vi "Acquisition Status.vi"(8 "error in (no error)":errorcluster, 9 "Remarks":string, 10 "Status":bool, 11 "Controller in":refnum<class "Controller.lvclass">) -> (0 "error out":errorcluster, 3 "Controller out":refnum<class "Controller.lvclass">)   [LabVIEW 2022 SP3, in "Controller.lvlib" / "Controller.lvclass"]
uses:
  Controller.lvclass
  Controller.lvclass/Controller.ctl
  UserInterface/UserInterface Messages/Log Data Msg/Log Data Msg.lvclass/Log Data Msg.ctl
  <vilib>/ActorFramework/Message Enqueuer/Message Enqueuer.lvclass/Message Enqueuer.ctl
  Read PLC-Handler Enqueuer.vi
  Read UI Enqueuer.vi
  <vilib>/ActorFramework/Message Enqueuer/Enqueue.vi
  UserInterface/UserInterface Messages/Log Data Msg/Log Data Msg.lvclass
  C:/Program Files/National Instruments/LabVIEW 2022/vi.lib/ActorFramework/Message/Message.lvclass
  PLCHandler/PLCHandler Messages/Acknowledgement Msg/Acknowledgement Msg.lvclass
  PLCHandler/PLCHandler Messages/Sleep Msg/Sleep Msg.lvclass
  <vilib>/ActorFramework/Message Priority Queue/Priority Enqueue.vi
  <vilib>/ActorFramework/Message Enqueuer/Message Enqueuer.lvclass
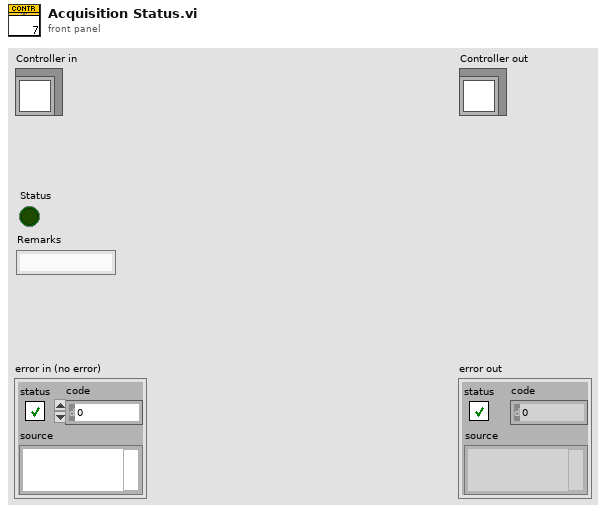
[diagram p1: front panel]
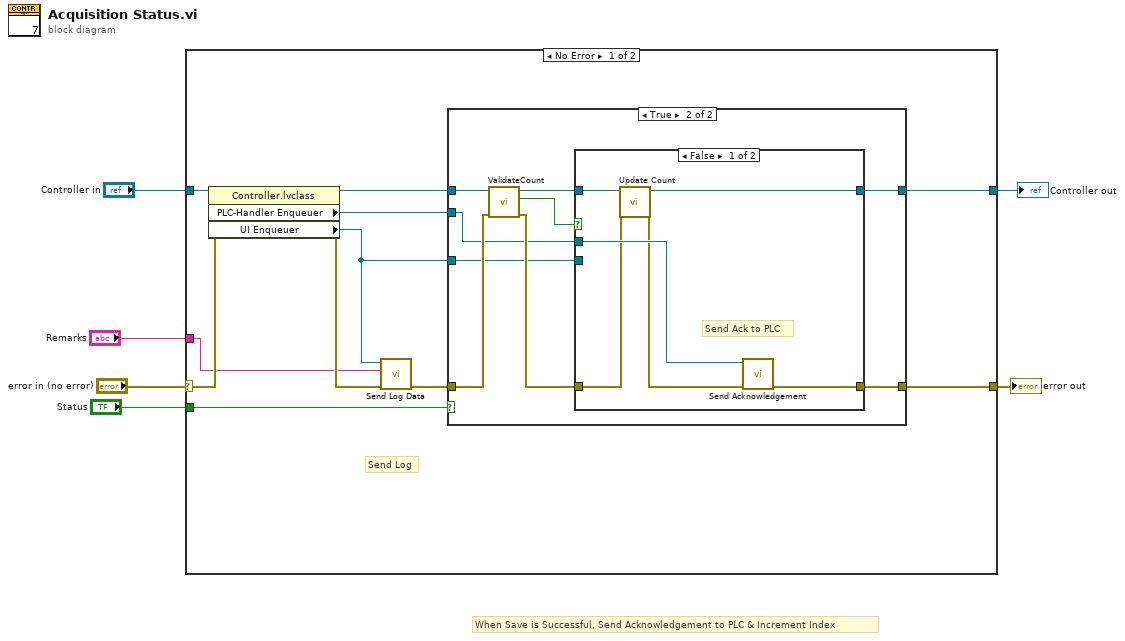
[diagram p0: block diagram]
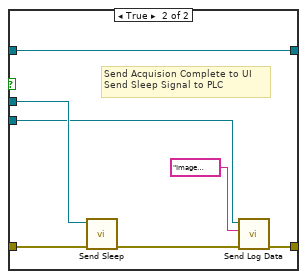
[diagram p3: hidden frame]
diagram:
  # "When Save is Successful, Send Acknowledgement to PLC & Increment Index"
  n1 = case shown="No Error" "error in (no error)" {
    selector: "error in (no error)" -> [w14 w42]
    tunnel: "Controller in" -> [w16 w43]
    tunnel: [w12 w43] -> w5
    tunnel: [w11 w42] -> w3
    tunnel: "Status" -> [w17 _]
    tunnel: "Remarks" -> [w7 _]
    frame No Error {
      # "Send Log"
      n2 = property class="Controller.lvclass"(reference=w16, error in=w14) -> (reference out=w13:refnum<class "Controller.lvclass">, error out=w9:errorcluster, "PLC-Handler Enqueuer"=w15:refnum<class "Message Enqueuer.lvclass">, "UI Enqueuer"=w10:refnum<class "Message Enqueuer.lvclass">)
      n3 = call "Send Log Data.vi"("error in (no error)"=w9, "Message"=w7, "Message Enqueuer"=w10) -> ("error out"=w8:errorcluster)  [unwired: 7 in, 1 out]
      n4 = case shown="True" w17 {
        tunnel: w8 -> [w18 w27]
        tunnel: w15 -> [_ w23]
        tunnel: w13 -> [w19 w28]
        tunnel: [w19 w21] -> w12
        tunnel: [w18 w24] -> w11
        tunnel: w10 -> [_ w20]
        frame False {
        }
        frame True {
          n5 = call "ValidateCount.vi"("error in (no error)"=w27, "Controller in"=w28) -> ("error out"=w25:errorcluster, "AcquisitionComplete?"=w26:bool, "Controller out"=w22:refnum<class "Controller.lvclass">)  [unwired: 7 in]
          n6 = case shown="False" w26 {
            tunnel: w25 -> [w30 w39]
            tunnel: [w33 w37] -> w24
            tunnel: w23 -> [w34 w40]
            tunnel: w22 -> [w32 w41]
            tunnel: [w31 w41] -> w21
            tunnel: w20 -> [_ w36]
            frame False {
              # "Send Ack to PLC"
              n7 = call "Update Count.vi"("error in (no error)"=w30, "Controller in"=w32) -> ("error out"=w29:errorcluster, "Controller out"=w31:refnum<class "Controller.lvclass">)  [unwired: 8 in]
              n8 = call "Send Acknowledgement.vi"("error in (no error)"=w29, "Message Enqueuer"=w34) -> ("error out"=w33:errorcluster)  [unwired: 8 in, 1 out]
            }
            frame True {
              # "Send Acquision Complete to UI\nSend Sleep Signal to PLC"
              n9 = call "Send Sleep.vi"("error in (no error)"=w39, "Message Enqueuer"=w40) -> ("error out"=w38:errorcluster)  [unwired: 8 in, 1 out]
              n10 = call "Send Log Data.vi"("error in (no error)"=w38, "Message"="Image Acquisition Completed...", "Message Enqueuer"=w36) -> ("error out"=w37:errorcluster)  [unwired: 7 in, 1 out]
            }
          }
        }
      }
    }
    frame Error {
    }
  }
  "error out" <- w3
  "Controller out" <- w5
